vi "Panel Set Window Title.vi"(8 "error in (no error)":errorcluster, 10 "Front Panel Window:Title(\"\")":string, 11 "Panel Control_Ref in":refnum<class "Panel Controller.lvclass">) -> (0 "error out":errorcluster, 3 "Panel Control_Ref out":refnum<class "Panel Controller.lvclass">)   [LabVIEW 2015, in "Panel Controller.lvclass"]
uses:
  Panel Controller.lvclass
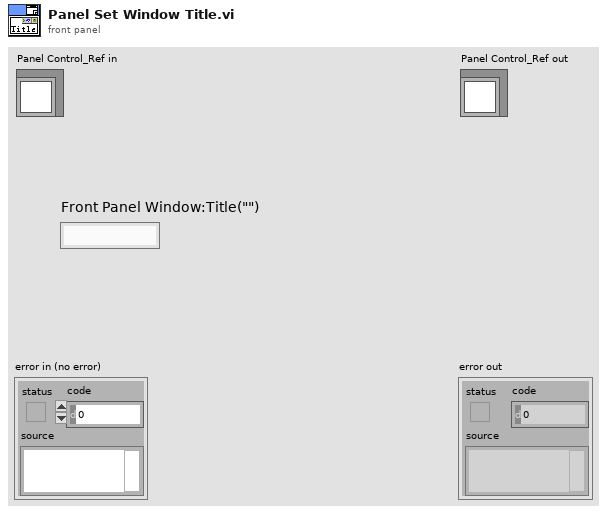
[diagram p1: front panel]
types:
  T1 = typedef "Panel Controller.lvclass/ObjectAttributes.ctl" = cluster{"Sub Panel Ref":refnum<vi>, "Panel_Q":refnum<queue>, "VI Running Refnum":refnum<vi>, "Brower Controller_Q":refnum<class "Message Enqueuer.lvclass">, "GUI Control Builder Director.lvclass":refnum<class "GUI Control Builder Director.lvclass">, "Panel GUI Manager.lvclass":refnum<class "Panel GUI Manager.lvclass">}
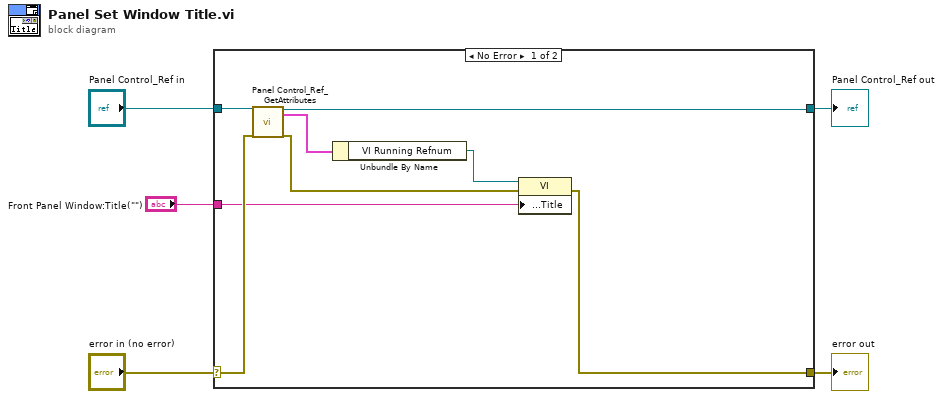
[diagram p0: block diagram]
diagram:
  n1 = case shown="No Error" "error in (no error)" {
    selector: "error in (no error)" -> [w12 w15]
    tunnel: [w7 w15] -> w4
    tunnel: [w6 w14] -> w2
    tunnel: "Panel Control_Ref in" -> [w13 w14]
    tunnel: "Front Panel Window:Title(\"\")" -> [w8 _]
    frame No Error {
      n2 = call "Panel Control_Ref_GetAttributes.vi"("reference in"=w13, "error in (no error)"=w12) -> ("reference out"=w6:refnum<class "Panel Controller.lvclass">, "Data"=w11:T1, "error out"=w9:errorcluster)  [unwired: 14 in, 1 out]
      n3 = Unbundle By Name(w11) -> ("VI Running Refnum"=w10:refnum<vi>)
      n4 = property class="VI"(reference=w10, error in=w9, "Front Panel.Title"=w8) -> (error out=w7:errorcluster)  [unwired: 1 out]
    }
    frame Error {
    }
  }
  "error out" <- w4
  "Panel Control_Ref out" <- w2
